vi "lab2.vi"() -> ()   [LabVIEW 2016]
panel:
  out "Hours":dbl
  out "Minutes":dbl
  out "Second":dbl
  out "Message":string
  out "Warning":bool
  in  "Total time in seconds":dbl
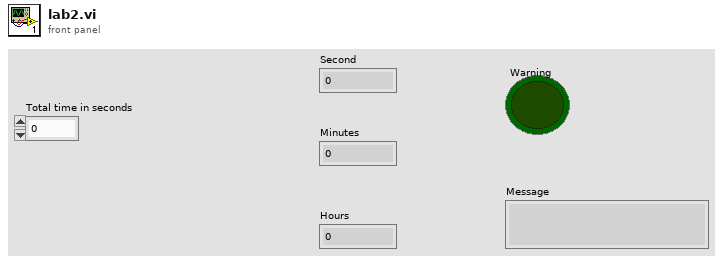
[diagram p1: front panel]
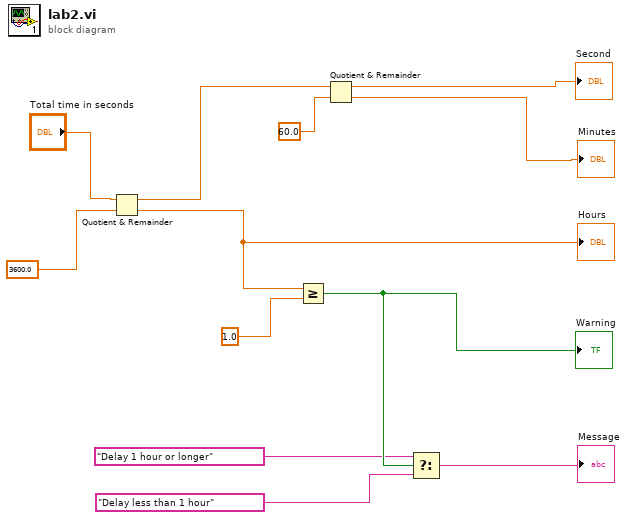
[diagram p0: block diagram]
diagram:
  n1 = Quotient & Remainder(x="Total time in seconds", y=3600.0) -> (x-y*floor(x/y)=w2:dbl, floor(x/y)=w1:dbl)
  "Hours" <- w1
  n2 = Greater Or Equal?(x=w1, y=1.0) -> (x >= y?=w9:bool)
  "Warning" <- w9
  n3 = Quotient & Remainder(x=w2, y=60.0) -> (x-y*floor(x/y)=→"Second":dbl, floor(x/y)=→"Minutes":dbl)
  n4 = Select(t="Delay 1 hour or longer", s=w9, f="Delay less than 1 hour") -> (s? t:f=→"Message":string)
